vi "scale manipulation.vi"(5 "scale fit":T1(ring), 7 "rescale":T2(ring), 9 "y-array":dbl[](array[numeric]), 10 "x-array":dbl[](array[numeric]), 11 "graph reference in":refnum<vi>) -> (3 "reference out":refnum<vi>)   [LabVIEW 2025]
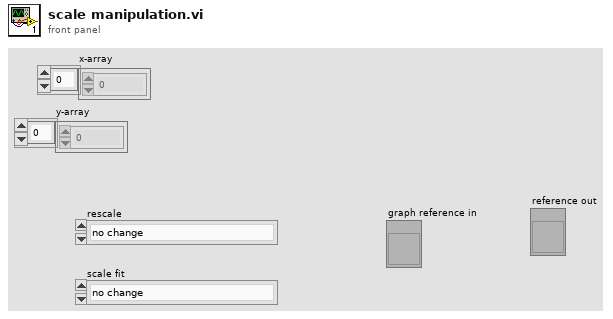
[diagram p1: front panel]
types:
  T1 = enum16{"no change", "no auto", "auto once", "auto"}
  T2 = enum16{"no change", "show whole data", "show whole panel"}
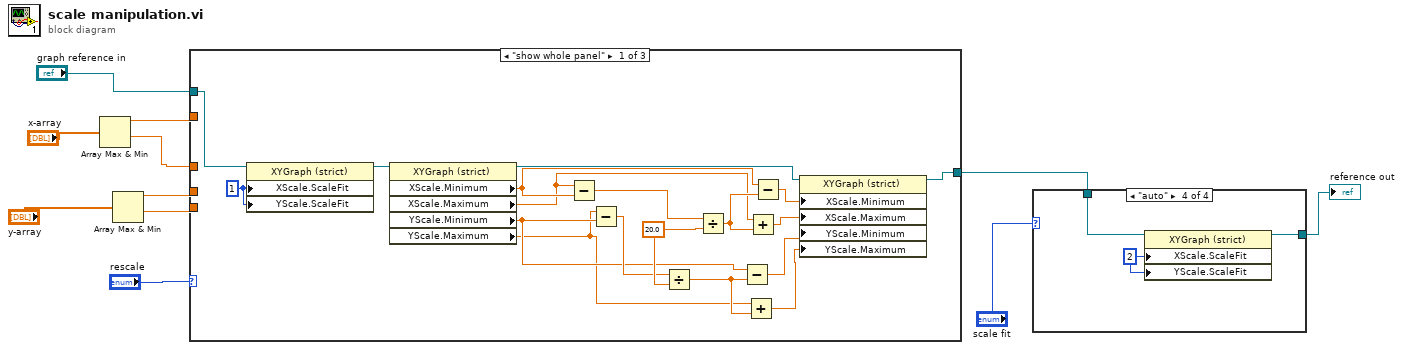
[diagram p0: block diagram]
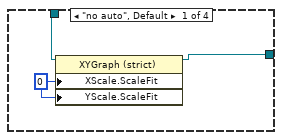
[diagram p2: hidden frame]
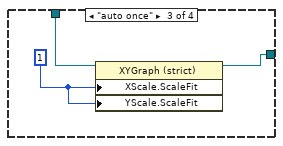
[diagram p4: hidden frame]
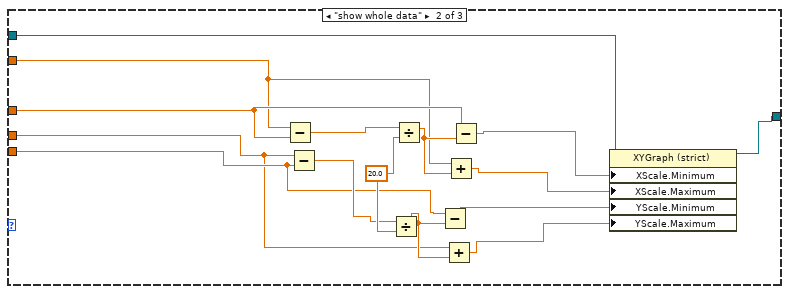
[diagram p5: hidden frame]
diagram:
  n1 = Array Max & Min(array="x-array") -> (max value=w7:dbl, min value=w8:dbl)  [unwired: 2 out]
  n2 = Array Max & Min(array="y-array") -> (max value=w5:dbl, min value=w6:dbl)  [unwired: 2 out]
  n3 = case shown="\"show whole panel\"" "rescale" {
    tunnel: w8 -> [_ w39 _]
    tunnel: w7 -> [_ w38 _]
    tunnel: w6 -> [_ w37 _]
    tunnel: w5 -> [_ w36 _]
    tunnel: "graph reference in" -> [w23 w31 w45]
    tunnel: [w12 w30 w45] -> w1
    frame "show whole panel" {
      w22 = u8 1 ("X Scale.Scale Fit")
      w28 = 20.0 ("y")
      n4 = property on="Property Node" class="XYGraph (strict)"(reference=w23, "XScale.ScaleFit"=w22, "YScale.ScaleFit"=w22) -> (reference out=w24:refnum<vi>)  [unwired: 1 in, 1 out]
      n5 = property on="Property Node" class="XYGraph (strict)"(reference=w24) -> (reference out=w17:refnum<vi>, "XScale.Minimum"=w21:dbl, "XScale.Maximum"=w20:dbl, "YScale.Minimum"=w19:dbl, "YScale.Maximum"=w18:dbl)  [unwired: 1 in, 1 out]
      n6 = Subtract(x=w20, y=w21) -> (x-y=w29:dbl)
      n7 = Subtract(x=w18, y=w19) -> (x-y=w27:dbl)
      n8 = Divide(x=w27, y=w28) -> (x/y=w25:dbl)
      n9 = Divide(x=w29, y=w28) -> (x/y=w26:dbl)
      n10 = Subtract(x=w19, y=w25) -> (x-y=w14:dbl)
      n11 = Add(x=w18, y=w25) -> (x+y=w13:dbl)
      n12 = Add(x=w20, y=w26) -> (x+y=w15:dbl)
      n13 = Subtract(x=w21, y=w26) -> (x-y=w16:dbl)
      n14 = property on="Property Node" class="XYGraph (strict)"(reference=w17, "XScale.Minimum"=w16, "XScale.Maximum"=w15, "YScale.Minimum"=w14, "YScale.Maximum"=w13) -> (reference out=w12:refnum<vi>)  [unwired: 1 in, 1 out]
    }
    frame "show whole data" {
      w43 = 20.0 ("y")
      n15 = Subtract(x=w38, y=w39) -> (x-y=w44:dbl)
      n16 = Subtract(x=w36, y=w37) -> (x-y=w42:dbl)
      n17 = Divide(x=w42, y=w43) -> (x/y=w40:dbl)
      n18 = Divide(x=w44, y=w43) -> (x/y=w41:dbl)
      n19 = Subtract(x=w37, y=w40) -> (x-y=w33:dbl)
      n20 = Add(x=w36, y=w40) -> (x+y=w32:dbl)
      n21 = Add(x=w38, y=w41) -> (x+y=w34:dbl)
      n22 = Subtract(x=w39, y=w41) -> (x-y=w35:dbl)
      n23 = property on="Property Node" class="XYGraph (strict)"(reference=w31, "XScale.Minimum"=w35, "XScale.Maximum"=w34, "YScale.Minimum"=w33, "YScale.Maximum"=w32) -> (reference out=w30:refnum<vi>)  [unwired: 1 in, 1 out]
    }
    frame "no change" {
    }
  }
  n24 = case shown="\"auto\"" "scale fit" {
    tunnel: [w46 w49 w51 w55] -> w9
    tunnel: w1 -> [w47 w49 w52 w53]
    frame "no auto", Default {
      w48 = u8 0 ("X Scale.Scale Fit")
      n25 = property on="Property Node" class="XYGraph (strict)"(reference=w47, "XScale.ScaleFit"=w48, "YScale.ScaleFit"=w48) -> (reference out=w46:refnum<vi>)  [unwired: 1 in, 1 out]
    }
    frame "no change" {
    }
    frame "auto once" {
      w50 = u8 1 ("X Scale.Scale Fit")
      n26 = property on="Property Node" class="XYGraph (strict)"(reference=w52, "XScale.ScaleFit"=w50, "YScale.ScaleFit"=w50) -> (reference out=w51:refnum<vi>)  [unwired: 1 in, 1 out]
    }
    frame "auto" {
      w54 = u8 2 ("X Scale.Scale Fit")
      n27 = property on="Property Node" class="XYGraph (strict)"(reference=w53, "XScale.ScaleFit"=w54, "YScale.ScaleFit"=w54) -> (reference out=w55:refnum<vi>)  [unwired: 1 in, 1 out]
    }
  }
  "reference out" <- w9
